vi "TCPIP.vi"() -> ()   [LabVIEW 2015]
uses:
  Galobal variable_TI.vi
panel:
  out "concatenated string":string
  in  "Client Closed":string="The client VI closed the connection."
  in  "Stop":bool
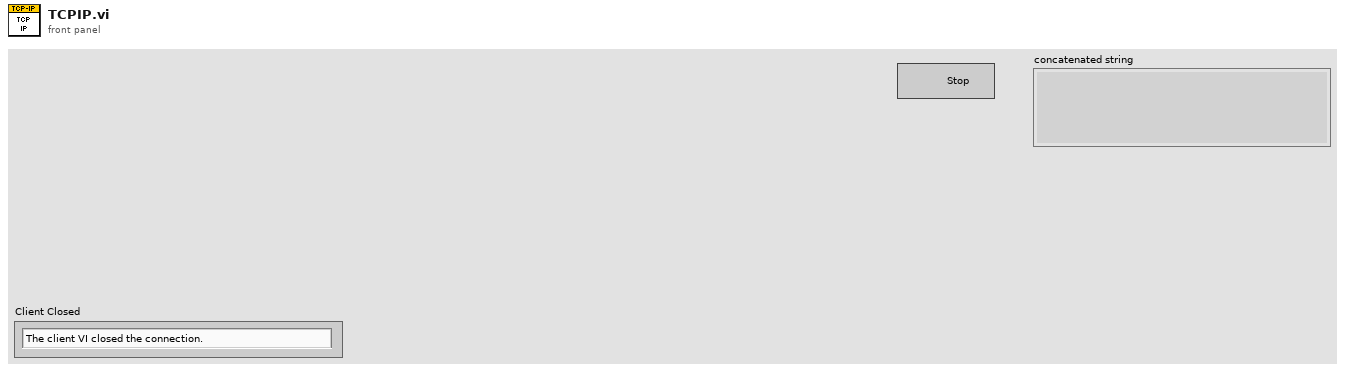
[diagram p1: front panel]
types:
  T1 = enum16{"Standard", "Buffered", "CRLF", "Immediate"}
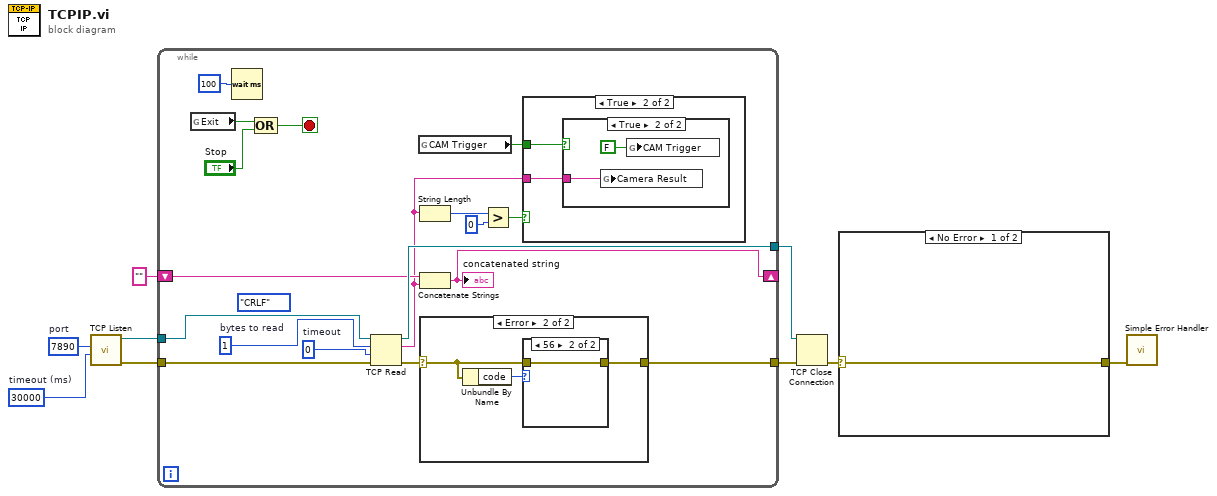
[diagram p0: block diagram]
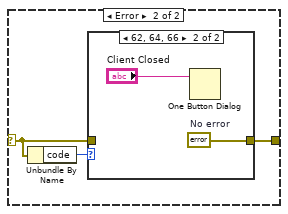
[diagram p2: hidden frame]
diagram:
  w2 = u16 7890  # port
  w3 = 30000  # timeout (ms)
  n1 = call <vilib>:"TCP Listen.vi"("timeout ms (wait forever: -1)"=w3, "port"=w2) -> ("error out"=w4:errorcluster, "connection ID"=w5:refnum<k5>)  [unwired: 5 in, 3 out]
  n2 = while {
    tunnel: [w21] -> w8
    tunnel: [w24] -> w9
    tunnel: w5 -> [w20]
    tunnel: w4 -> [w19]
    shift-right: [w15] -> _
    shift-left: "" -> [w16]
    stop <- w26 stop-if-true
    (unwired) T1."CRLF" ("mode (standard)")
    w23 = 0  # timeout
    w25 = 1  # bytes to read
    # "TCP Server Loop"
    n3 = global read "Galobal variable_TI.vi" "Exit"() -> (w11:bool)
    n4 = Wait (ms)(milliseconds to wait=u32 100) -> ()  [unwired: 1 out]
    n5 = Compound Arithmetic op=OR(w11, "Stop") -> (w26:bool)
    n6 = TCP Read(connection ID=w20, bytes to read=w25, error in (no error)=w19, 9:w23) -> (connection ID out=w24:refnum<k5>, data out=w10:string, error out=w22:errorcluster)  [unwired: 1 out]
    n7 = global read "Galobal variable_TI.vi" "CAM Trigger"() -> (w17:bool)
    n8 = String Length(string=w10) -> (length=w14:i32)
    n9 = Concatenate Strings(w16, w10) -> (w15:string)
    "concatenated string" <- w15
    n10 = case shown="Error" w22 {
      selector: w22 -> [w32 w34]
      tunnel: [w32 w33] -> w21
      frame No Error {
      }
      frame Error {
        n11 = Unbundle By Name(w34) -> ("code"=w35:i32)
        n12 = case shown="56" w35 {
          tunnel: w34 -> [w36 w37]
          tunnel: [w36 w37] -> w33
          frame Default {
          }
          frame 56 {
          }
        }
      }
    }
    n13 = Greater?(x=w14, y=0) -> (0:w12:bool)
    n14 = case shown="True" w12 {
      tunnel: w17 -> [_ w29]
      tunnel: w10 -> [_ w28]
      frame False {
      }
      frame True {
        n15 = case shown="True" w29 {
          tunnel: w28 -> [_ w31]
          frame False {
          }
          frame True {
            n16 = global write "Galobal variable_TI.vi" "Camera Result"(w31) -> ()
            n17 = global write "Galobal variable_TI.vi" "CAM Trigger"(FALSE ("CAM Trigger")) -> ()
          }
        }
      }
    }
  }
  n18 = TCP Close Connection(connection ID=w9, error in (no error)=w8) -> (error out=w7:errorcluster)  [unwired: 2 out]
  n19 = case shown="No Error" w7 {
    selector: w7 -> [w38 w40]
    tunnel: [w38 w39] -> w6
    frame No Error {
    }
    frame Error {
      n20 = Unbundle By Name(w40) -> ("code"=w41:i32)
      n21 = case shown="62, 64, 66" w41 {
        tunnel: w40 -> [w42 _]
        tunnel: [w42 w44] -> w39
        frame Default {
        }
        frame 62, 64, 66 {
          w44 = errorcluster {"status"=FALSE, "code"=0, "source"=""}  # No error
          n22 = One Button Dialog(message="Client Closed") -> ()  [unwired: 1 in, 1 out]
        }
      }
    }
  }
  n23 = call <vilib>:"Simple Error Handler.vi"("error in (no error)"=w6) -> ()  [unwired: 1 in, 8 out]
